vi "RefnameToString.vi"(1 "Enum":T1) -> (0 "Refname":string)   [LabVIEW 2014]
uses:
  Refname.ctl
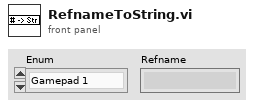
[diagram p1: front panel]
types:
  T1 = typedef "Refname.ctl" = enum16{"Gamepad 1", "Gamepad 2", "Drive Motors", "Strafe Motor", "Arm Clapper Motor", "Arm Angle", "Arm Belt Left", "Arm Belt Right", "Elevator 1", "Elevator 2", "Wiper"}
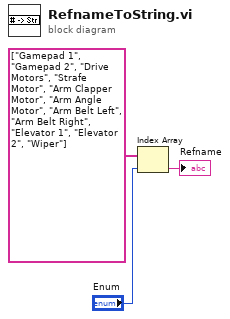
[diagram p0: block diagram]
diagram:
  n1 = Index Array(array=string[] ["Gamepad 1", "Gamepad 2", "Drive Motors", "Strafe Motor", "Arm Clapper Motor", "Arm Angle Motor", "Arm Belt Left", "Arm Belt Right", "Elevator 1", "Elevator 2", "Wiper"], index="Enum") -> (element=→"Refname":string)
